vi "Get Value (Bool).vi"(8 "error in":errorcluster, 11 "Sub Obj in":refnum<class "Sub Object.lvclass">) -> (0 "error out":errorcluster, 2 "Value":bool, 3 "Sub Obj out":refnum<class "Sub Object.lvclass">)   [LabVIEW 2020, in "CANopen.lvlib" / "Sub Object.lvclass"]
uses:
  Sub Object.lvclass
  Sub Object.lvclass/Sub Object.ctl
  Typedefs/Data Type.ctl
  CANopen.lvlib
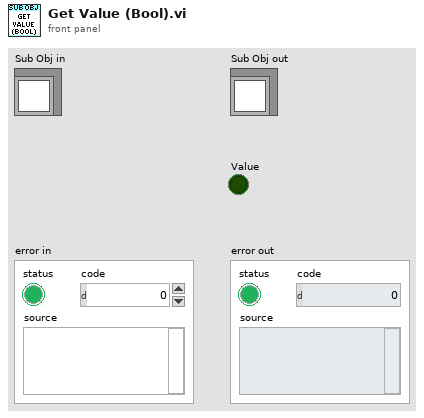
[diagram p1: front panel]
types:
  T1 = typedef "CANopen.lvlib/Data Type.ctl" = u16
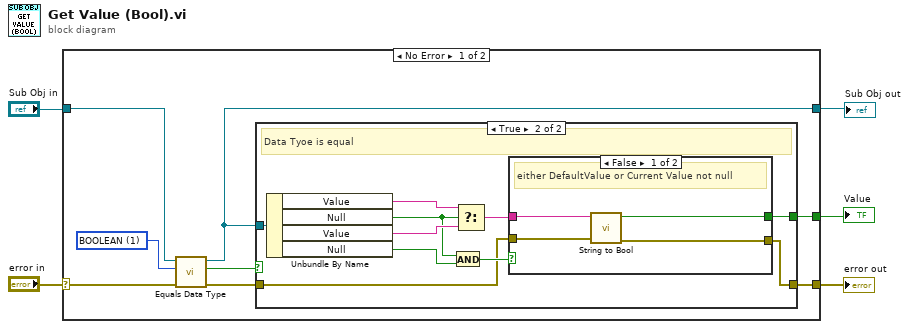
[diagram p0: block diagram]
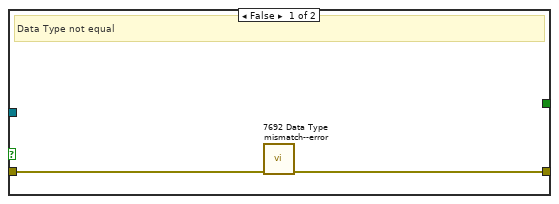
[diagram p2: hidden frame]
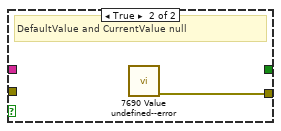
[diagram p3: hidden frame]
diagram:
  n1 = case shown="No Error" "error in" {
    selector: "error in" -> [w11 w32]
    tunnel: [w13 w32] -> w1
    tunnel: [w8 w31] -> w3
    tunnel: "Sub Obj in" -> [w9 w31]
    tunnel: [w12 _] -> w2
    frame No Error {
      w7 = T1 1 items=["BOOLEAN"=1, "INTEGER8"=2, "INTEGER16"=3, "INTEGER32"=4, "UNSIGNED8"=5, "UNSIGNED16"=6, "UNSIGNED32"=7, "REAL32"=8, "VISIBLE_STRING"=9, "OCTET_STRING"=10, "UNICODE_STRING"=11, "TIME_OF_DAY"=12, "TIME_DIFFERENCE"=13, "RESERVED1"=14, "DOMAIN"=15, "INTEGER24"=16, "REAL64"=17, "INTEGER40"=18, "INTEGER48"=19, "INTEGER56"=20, "INTEGER64"=21, "UNSIGNED24"=22, "RESERVED2"=23, "UNSIGNED40"=24, "UNSIGNED48"=25, "UNSIGNED56"=26, "UNSIGNED64"=27, "RESERVED3"=28, "RESERVED4"=29, "RESERVED5"=30, "RESERVED6"=31, "PDO_COMMUNICATION_PARAMETER"=32, "PDO_MAPPING"=33, "SDO_PARAMETER"=34, "IDENTITY"=35, "RESERVED7"=36] ("Data Type")
      n2 = call "Equals Data Type.vi"("error in"=w11, "Data Type"=w7, "Sub Obj in"=w9) -> ("error out"=w10:errorcluster, "Equal"=w6:bool, "Sub Obj out"=w8:refnum<class "Sub Object.lvclass">)  [unwired: 6 in]
      n3 = case shown="True" w6 {
        tunnel: w8 -> [_ w19]
        tunnel: [w14 w18] -> w13
        tunnel: [_ w17] -> w12
        tunnel: w10 -> [w15 w16]
        frame False {
          # "Data Type not equal"
          n4 = call "7692 Data Type mismatch--error.vi"("error in"=w15) -> ("error out"=w14:errorcluster)  [unwired: 9 in, 1 out]
        }
        frame True {
          # "Data Tyoe is equal"
          n5 = Unbundle By Name(w19) -> ("Value"=w25:string, "Null"=w21:bool, "Value"=w23:string, "Null"=w22:bool)
          n6 = And(x=w21, y=w22) -> (x .and. y?=w20:bool)
          n7 = Select(t=w25, s=w21, f=w23) -> (s? t:f=w24:string)
          n8 = case shown="False" w20 {
            tunnel: [w28 w30] -> w18
            tunnel: w24 -> [w29 _]
            tunnel: [w27 _] -> w17
            tunnel: w16 -> [w26 _]
            frame False {
              # "either DefaultValue or Current Value not null"
              n9 = call "String to Bool.vi"("error in"=w26, "Integer String"=w29) -> ("error out"=w28:errorcluster, "Bool"=w27:bool)  [unwired: 8 in]
            }
            frame True {
              # "DefaultValue and CurrentValue null"
              n10 = call "7690 Value undefined--error.vi"() -> ("error out"=w30:errorcluster)  [unwired: 10 in, 1 out]
            }
          }
        }
      }
    }
    frame Error {
    }
  }
  "Sub Obj out" <- w3
  "error out" <- w1
  "Value" <- w2
